vi "StartServerVi.vi"(0 "Baxter":T2) -> (1 "Active Topics":T1(array[cluster]), 2 "Reply":string, 3 "Baxter out":T2)   [LabVIEW 2013]
uses:
  _ROSControl.ctl
  _ROSDirection.ctl
  _ROSDefinition.vi
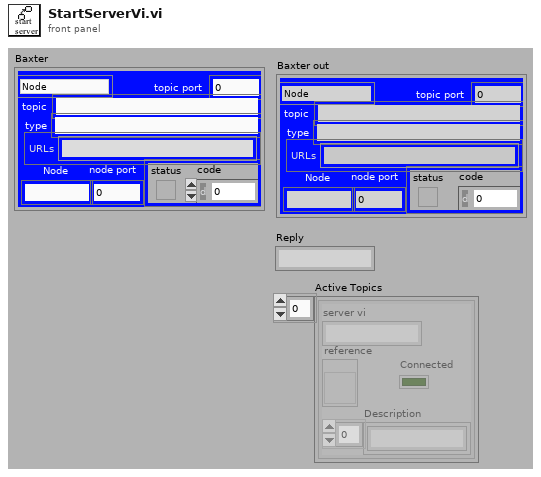
[diagram p1: front panel]
types:
  T1 = cluster{"server vi":string, "reference":refnum<vi>, "Description":string[], "Connected":bool}[]
  T2 = typedef "_ROSControl.ctl" = cluster{"topic port":u16, "Node":string, "topic":string, "type":string, "node port":u32, "error ":errorcluster, "Direction":T3, "APIs":string[]}
  T3 = typedef "_ROSDirection.ctl" = enum16{"Node", "Publisher", "Subscriber", "Service Client"}
  T4 = enum32{"Bad", "Idle", "Run top level", "Running"}
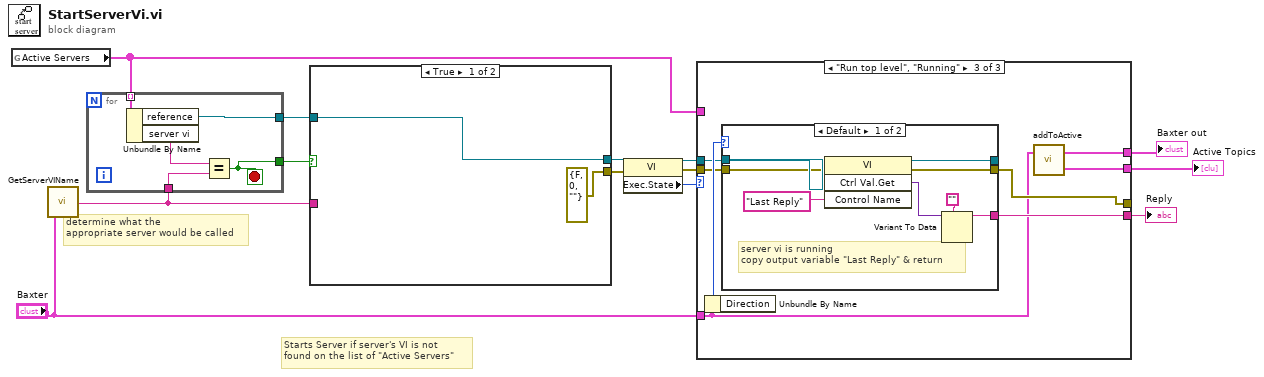
[diagram p0: block diagram]
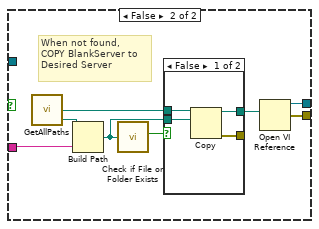
[diagram p2: hidden frame]
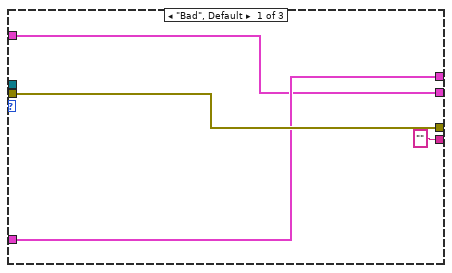
[diagram p4: hidden frame]
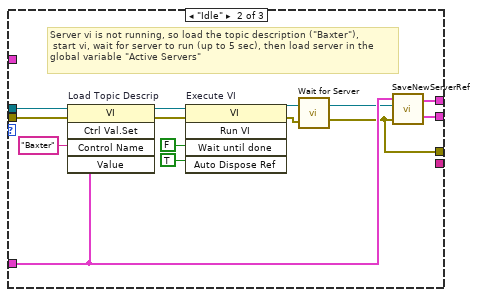
[diagram p5: hidden frame]
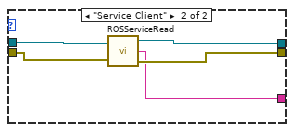
[diagram p6: hidden frame]
diagram:
  # "Starts Server if server's VI is not\nfound on the list of \"Active Servers\""
  # "determine what the \nappropriate server would be called"
  n1 = global read "_ROSDefinition.vi" "Active Servers"() -> (w1:T1)
  n2 = call "GetServerVIName.vi"("Baxter"="Baxter") -> ("vi name"=w5:string)
  n3 = for {
    tunnel: w1 -> [w18] mode=indexing
    tunnel: w5 -> [w16]
    tunnel: [w15] -> w4
    tunnel: [w14] -> w3
    stop <- w15 stop-if-true
    n4 = Unbundle By Name(w18) -> ("reference"=w14:refnum<vi>, "server vi"=w17:string)
    n5 = Equal?(x=w17, y=w16) -> (x = y?=w15:bool)
  }
  n6 = case shown="True" w4 {
    tunnel: w5 -> [_ w28]
    tunnel: [w19 w22] -> w12
    tunnel: [errorcluster {"status"=FALSE, "code"=0, "source"=""} ("error out") w21] -> w11
    tunnel: w3 -> [w19 _]
    frame True {
    }
    frame False {
      # "When not found,\nCOPY BlankServer to\nDesired Server"
      n7 = call "GetAllPaths.vi"() -> ("Server Folder"=w23:path, "BlankServer"=w24:path)  [unwired: 1 in, 1 out]
      n8 = Build Path(base path=w23, name or relative path=w28) -> (appended path=w26:path)
      n9 = call <vilib>:"Check if File or Folder Exists.vi"("path"=w26) -> ("file or folder exists?"=w25:bool)  [unwired: 8 in, 2 out]
      n10 = case shown="False" w25 {
        tunnel: w24 -> [w32 _]
        tunnel: w26 -> [w31 w33]
        tunnel: [w30 w33] -> w27
        tunnel: [w29 _] -> _
        frame False {
          n11 = Copy(10:w31, 11:w32) -> (0:w29:errorcluster, 3:w30:path)  [unwired: 3 in, 1 out]
        }
        frame True {
        }
      }
      n12 = Open VI Reference(vi path=w27) -> (vi reference=w22:refnum<vi>, error out=w21:errorcluster)  [unwired: 5 in]
    }
  }
  n13 = property class="VI"(reference=w12, error in=w11) -> (reference out=w9:refnum<vi>, error out=w8:errorcluster, "Exec.State"=w10:T4)
  n14 = case shown="\"Run top level\", \"Running\"" w10 {
    tunnel: w9 -> [_ w49 w58]
    tunnel: [w37 w41 w56] -> _
    tunnel: w8 -> [w37 w46 w57]
    tunnel: "Baxter" -> [w35 w45 w52]
    tunnel: ["" ("Control Name") _ w55] -> w13
    tunnel: [w35 w44 w53] -> w6
    tunnel: [w34 w43 w54] -> w2
    tunnel: w1 -> [w34 _ _]
    frame "Bad", Default {
    }
    frame "Idle" {
      # "Server vi is not running, so load the topic description (\"Baxter\"),\n start vi, wait for server to run (up to 5 sec), then load server in the \nglobal variable \"Active Servers\""
      n15 = invoke on="Load Topic Descrip" class="VI" method="Ctrl Val.Set"(reference=w49, error in=w46, "Control Name"="Baxter", "Value"=w45) -> (reference out=w48:refnum<vi>, error out=w38:errorcluster)  [unwired: 1 in, 3 out]
      n16 = invoke on="Execute VI" class="VI" method="Run VI"(reference=w48, error in=w38, "Wait until done"=FALSE ("Wait Until Done"), "Auto Dispose Ref"=TRUE ("Wait Until Done")) -> (reference out=w39:refnum<vi>, error out=w40:errorcluster)  [unwired: 1 in, 3 out]
      n17 = call "Wait for Server.vi"("error in"=w40, "vi reference in"=w39) -> ("error out"=w41:errorcluster, "vi reference out"=w42:refnum<vi>)  [unwired: 1 out]
      n18 = call "SaveNewServerRef.vi"("error"=w41, "vi reference"=w42, "Baxter in"=w45) -> ("Active Topics"=w43:T1, "Baxter out"=w44:T2)
    }
    frame "Run top level", "Running" {
      n19 = Unbundle By Name(w52) -> ("Direction"=w59:T3)
      n20 = case shown="Default" w59 {
        tunnel: w58 -> [w64 w72]
        tunnel: w57 -> [w65 w69]
        tunnel: [w62 w71] -> _
        tunnel: [w63 w70] -> w56
        tunnel: [w60 w68] -> w55
        frame Default {
          # "server vi is running\ncopy output variable \"Last Reply\" & return"
          n21 = invoke class="VI" method="Ctrl Val.Get"(reference=w64, error in=w65, "Control Name"="Last Reply") -> (reference out=w62:refnum<vi>, error out=w63:errorcluster, "Get Control Value Variant"=w66:variant)  [unwired: 1 in, 1 out]
          n22 = Variant To Data(type="" ("Control Name"), Variant=w66) -> (data=w60:string)  [unwired: 1 in, 1 out]
        }
        frame "Service Client" {
          n23 = call "ROSServiceRead.vi"("error in"=w69, "vi reference"=w72) -> ("error out"=w70:errorcluster, "Reply"=w68:string, "vi reference"=w71:refnum<vi>)
        }
      }
      n24 = call "addToActive.vi"("Baxter in"=w52) -> ("Active Topics"=w54:T1, "Baxter out"=w53:T2)  [unwired: 1 in]
    }
  }
  "Baxter out" <- w6
  "Reply" <- w13
  "Active Topics" <- w2
